vi "SQLPrepare.vi"(4 "error in (no error)":errorcluster, 6 "StatementText":string, 7 "InputHandle":i32) -> (0 "error out":errorcluster, 3 "OutputHandle":i32)   [LabVIEW 2011]
doc: "Charge la requête spécifiée par le lien, ceci sans l'exécuter"
uses:
  Odbc32.dll
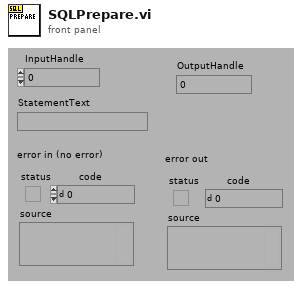
[diagram p1: front panel]
types:
  T1 = enum16{"NOPE", "SQL_HANDLE_ENV", "SQL_HANDLE_DBC", "SQL_HANDLE_STMT", "SQL_HANDLE_DESC"}
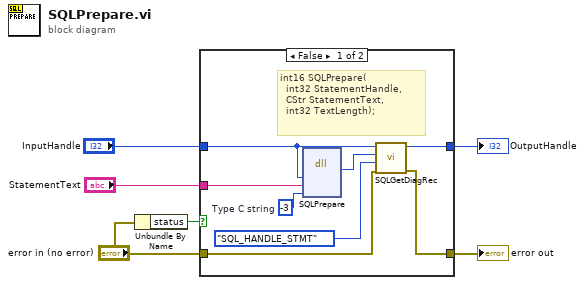
[diagram p0: block diagram]
diagram:
  n1 = Unbundle By Name("error in (no error)") -> ("status"=w1:bool)
  n2 = case shown="False" w1 {
    tunnel: "StatementText" -> [w14 _]
    tunnel: "InputHandle" -> [w12 w15]
    tunnel: [w11 w15] -> w4
    tunnel: "error in (no error)" -> [w9 w16]
    tunnel: [w8 w16] -> w3
    frame False {
      w13 = -3  # Type C string
      # "int16 SQLPrepare(\n  int32 StatementHandle, \n  CStr StatementText, \n  int32 TextLength);"
      n3 = dll-call lib="Odbc32.dll" fn="SQLPrepare"("StatementHandle"=w12, "StatementText"=w14, "TextLength"=w13) -> (w10:i16)  [unwired: 6 in, 2 out]
      n4 = call "SQLGetDiagRec.vi"("error in (no error)"=w9, "HandleType"=T1."SQL_HANDLE_STMT", "Status (SQL_SUCCESS=0)"=w10, "Input Handle"=w12) -> ("error out"=w8:errorcluster, "Output Handle"=w11:i32)  [unwired: 2 out]
    }
    frame True {
    }
  }
  "OutputHandle" <- w4
  "error out" <- w3
